vi "tsapp_transmit_canfd_sync.vi"(8 "error in (no error)":errorcluster, 9 "ATimeoutMS":i32, 10 "TCANFD":T1 {"ADLC" items=["0", "1", "2", "3", "4", "5", "6", "7", "8", "12", "16", "20", "24", "32", "48", "64"]; "AIsData" items=["Data Frame", "Remote Frame"]; "AIsStd" items=["标准帧", "扩展帧"]; "AId" format="%x"; "AIdxchn" items=["CHN1", "CHN2", "CHN3", "CHN4", "CHN5", "CHN6", "CHN7", "CHN8", "CHN9", "CHN10", "CHN11", "CHN12", "CHN13", "CHN14", "CHN15", "CHN16", "CHN17", "CHN18", "CHN19", "CHN20", "CHN21", "CHN22", "CHN23", "CHN24", "CHN25", "CHN26", "CHN27", "CHN28", "CHN29", "CHN30", "CHN31", "CHN32"]}, 11 "Path":path) -> (0 "error out":errorcluster, 2 "return":i32, 3 "Path output":path)   [LabVIEW 2014]
doc: "Function Introduction :\nSend CANFD message and only exit this function after detecting successful transmission. This function returns success,\nThe CANFD message must have been successfully sent to the CAN bus.\nCall location :\nSend CANFD message\nlimitations\nBecause this function requires deep support for device APIs, currently only TS supports this function interface\nAnd Vector series devices.\ninput parameter :\nACANFD: CANFD data packet. Please refer to chapter: TLIBCANFD: CANFD for the composition of TLIBCANFD data\nData type.\nATimeoutMS: timeout (milliseconds)\nReturn value :\n==0: Sent successfully\nOther values: Sending failed, please refer to the error code for the reason of the failure"
uses:
  Typedef/TLibCANFD_Interface.ctl
  Typedef/TLibCANFD.ctl
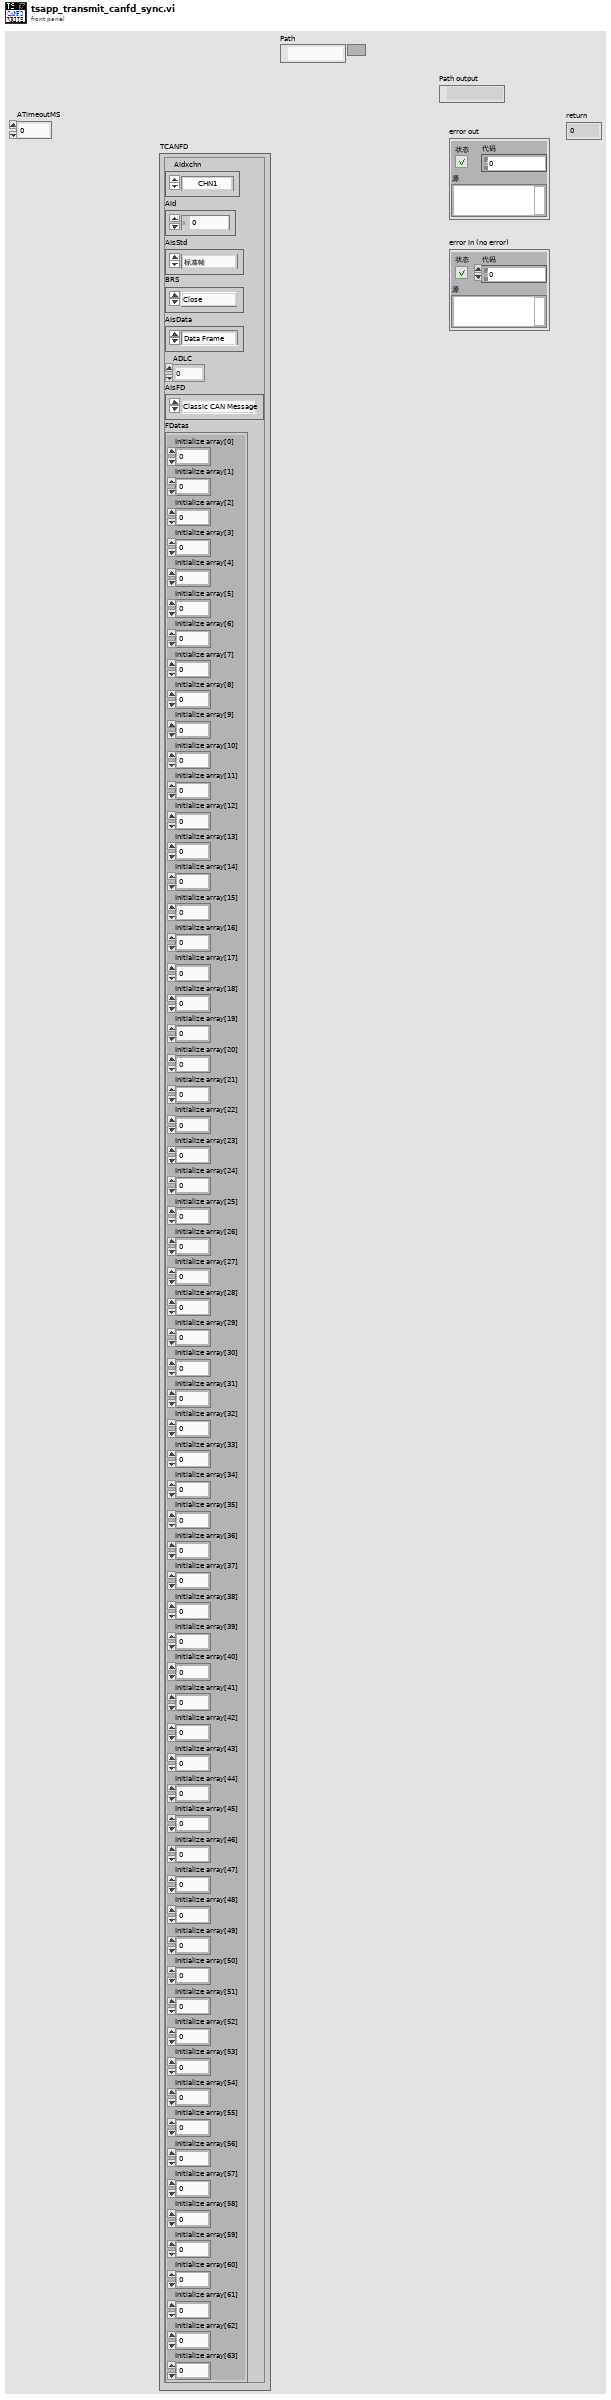
[diagram p1: front panel]
types:
  T1 = typedef "TLibCANFD.ctl" = cluster{"AIdxchn":u8, "AId":i32, "AIsStd":u8, "BRS":enum16{"Close", "Open"}, "AIsData":u8, "ADLC":i32, "AIsFD":enum16{"Classic CAN Message", "FD CAN Message"}, "FDatas":cluster{"Initialize array[0]":u8, "Initialize array[1]":u8, "Initialize array[2]":u8, "Initialize array[3]":u8, "Initialize array[4]":u8, "Initialize array[5]":u8, "Initialize array[6]":u8, "Initialize array[7]":u8, "Initialize array[8]":u8, "Initialize array[9]":u8, "Initialize array[10]":u8, "Initialize array[11]":u8, "Initialize array[12]":u8, "Initialize array[13]":u8, "Initialize array[14]":u8, "Initialize array[15]":u8, "Initialize array[16]":u8, "Initialize array[17]":u8, "Initialize array[18]":u8, "Initialize array[19]":u8, "Initialize array[20]":u8, "Initialize array[21]":u8, "Initialize array[22]":u8, "Initialize array[23]":u8, "Initialize array[24]":u8, "Initialize array[25]":u8, "Initialize array[26]":u8, "Initialize array[27]":u8, "Initialize array[28]":u8, "Initialize array[29]":u8, "Initialize array[30]":u8, "Initialize array[31]":u8, "Initialize array[32]":u8, "Initialize array[33]":u8, "Initialize array[34]":u8, "Initialize array[35]":u8, "Initialize array[36]":u8, "Initialize array[37]":u8, "Initialize array[38]":u8, "Initialize array[39]":u8, "Initialize array[40]":u8, "Initialize array[41]":u8, "Initialize array[42]":u8, "Initialize array[43]":u8, "Initialize array[44]":u8, "Initialize array[45]":u8, "Initialize array[46]":u8, "Initialize array[47]":u8, "Initialize array[48]":u8, "Initialize array[49]":u8, "Initialize array[50]":u8, "Initialize array[51]":u8, "Initialize array[52]":u8, "Initialize array[53]":u8, "Initialize array[54]":u8, "Initialize array[55]":u8, "Initialize array[56]":u8, "Initialize array[57]":u8, "Initialize array[58]":u8, "Initialize array[59]":u8, "Initialize array[60]":u8, "Initialize array[61]":u8, "Initialize array[62]":u8, "Initialize array[63]":u8}}
  T2 = typedef "TLibCANFD_Interface.ctl" = cluster{"FIdxChn":u8, "FProperties":u8, "FDLC":u8, "FFDProperties":u8, "FIdentifier":i32, "FTimeUS":u64, "FData":cluster{"[0]":u8, "[1]":u8, "[2]":u8, "[3]":u8, "[4]":u8, "[5]":u8, "[6]":u8, "[7]":u8, "[8]":u8, "[9]":u8, "[10]":u8, "[11]":u8, "[12]":u8, "[13]":u8, "[14]":u8, "[15]":u8, "[16]":u8, "[17]":u8, "[18]":u8, "[19]":u8, "[20]":u8, "[21]":u8, "[22]":u8, "[23]":u8, "[24]":u8, "[25]":u8, "[26]":u8, "[27]":u8, "[28]":u8, "[29]":u8, "[30]":u8, "[31]":u8, "[32]":u8, "[33]":u8, "[34]":u8, "[35]":u8, "[36]":u8, "[37]":u8, "[38]":u8, "[39]":u8, "[40]":u8, "[41]":u8, "[42]":u8, "[43]":u8, "[44]":u8, "[45]":u8, "[46]":u8, "[47]":u8, "[48]":u8, "[49]":u8, "[50]":u8, "[51]":u8, "[52]":u8, "[53]":u8, "[54]":u8, "[55]":u8, "[56]":u8, "[57]":u8, "[58]":u8, "[59]":u8, "[60]":u8, "[61]":u8, "[62]":u8, "[63]":u8}}
  T3 = cluster{"Initialize array[0]":u8, "Initialize array[1]":u8, "Initialize array[2]":u8, "Initialize array[3]":u8, "Initialize array[4]":u8, "Initialize array[5]":u8, "Initialize array[6]":u8, "Initialize array[7]":u8, "Initialize array[8]":u8, "Initialize array[9]":u8, "Initialize array[10]":u8, "Initialize array[11]":u8, "Initialize array[12]":u8, "Initialize array[13]":u8, "Initialize array[14]":u8, "Initialize array[15]":u8, "Initialize array[16]":u8, "Initialize array[17]":u8, "Initialize array[18]":u8, "Initialize array[19]":u8, "Initialize array[20]":u8, "Initialize array[21]":u8, "Initialize array[22]":u8, "Initialize array[23]":u8, "Initialize array[24]":u8, "Initialize array[25]":u8, "Initialize array[26]":u8, "Initialize array[27]":u8, "Initialize array[28]":u8, "Initialize array[29]":u8, "Initialize array[30]":u8, "Initialize array[31]":u8, "Initialize array[32]":u8, "Initialize array[33]":u8, "Initialize array[34]":u8, "Initialize array[35]":u8, "Initialize array[36]":u8, "Initialize array[37]":u8, "Initialize array[38]":u8, "Initialize array[39]":u8, "Initialize array[40]":u8, "Initialize array[41]":u8, "Initialize array[42]":u8, "Initialize array[43]":u8, "Initialize array[44]":u8, "Initialize array[45]":u8, "Initialize array[46]":u8, "Initialize array[47]":u8, "Initialize array[48]":u8, "Initialize array[49]":u8, "Initialize array[50]":u8, "Initialize array[51]":u8, "Initialize array[52]":u8, "Initialize array[53]":u8, "Initialize array[54]":u8, "Initialize array[55]":u8, "Initialize array[56]":u8, "Initialize array[57]":u8, "Initialize array[58]":u8, "Initialize array[59]":u8, "Initialize array[60]":u8, "Initialize array[61]":u8, "Initialize array[62]":u8, "Initialize array[63]":u8}
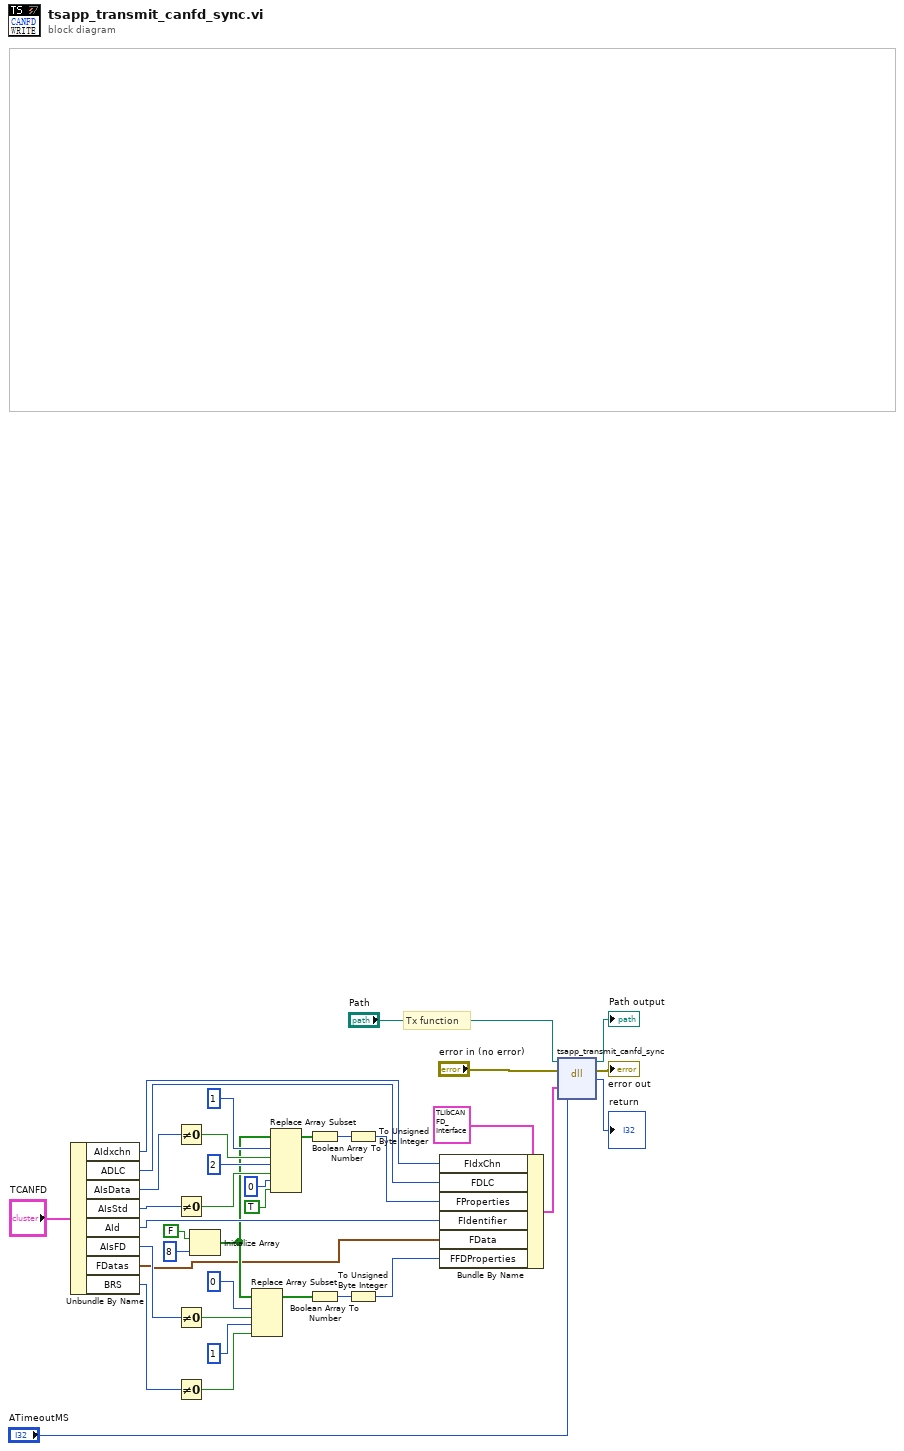
[diagram p0: block diagram]
diagram:
  # "Tx function"
  n1 = Unbundle By Name("TCANFD") -> ("AIdxchn"=w29:u8, "ADLC"=w20:i32, "AIsData"=w28:u8, "AIsStd"=w27:u8, "AId"=w30:i32, "AIsFD"=w15:enum16{"Classic CAN Message", "FD CAN Message"}, "FDatas"=w3:T3, "BRS"=w5:enum16{"Close", "Open"})
  n2 = Not Equal To 0?(x=w28) -> (x != 0?=w25:bool)
  n3 = Not Equal To 0?(x=w27) -> (x != 0?=w23:bool)
  n4 = Not Equal To 0?(x=w15) -> (x != 0?=w14:bool)
  n5 = Not Equal To 0?(x=w5) -> (x != 0?=w4:bool)
  n6 = Initialize Array(FALSE, 8 ("维数大小")) -> (w9:bool[])
  n7 = Replace Array Subset(array=w9, new element #1=w14, index #1=0 ("索引"), new element #2=w4, index #2=1 ("索引")) -> (w16:bool[])
  n8 = Replace Array Subset(array=w9, new element #1=w25, index #1=1 ("索引"), new element #2=w23, index #2=2 ("索引"), new element #3=TRUE ("新元素/子数组"), index #3=0 ("索引")) -> (w22:bool[])
  n9 = Boolean Array To Number(Boolean array=w22) -> (number=w21:u32)
  n10 = Boolean Array To Number(Boolean array=w16) -> (number=w17:u32)
  n11 = To Unsigned Byte Integer(number=w21) -> (unsigned 8bit integer=w19:u8)
  n12 = To Unsigned Byte Integer(number=w17) -> (unsigned 8bit integer=w12:u8)
  n13 = Bundle By Name(cluster=T2 {"FIdxChn"=0, "FProperties"=0, "FDLC"=0, "FFDProperties"=0, "FIdentifier"=0, "FTimeUS"=0, "FData"={"[0]"=0, "[1]"=0, "[2]"=0, "[3]"=0, "[4]"=0, "[5]"=0, "[6]"=0, "[7]"=0, "[8]"=0, "[9]"=0, "[10]"=0, "[11]"=0, "[12]"=0, "[13]"=0, "[14]"=0, "[15]"=0, "[16]"=0, "[17]"=0, "[18]"=0, "[19]"=0, "[20]"=0, "[21]"=0, "[22]"=0, "[23]"=0, "[24]"=0, "[25]"=0, "[26]"=0, "[27]"=0, "[28]"=0, "[29]"=0, "[30]"=0, "[31]"=0, "[32]"=0, "[33]"=0, "[34]"=0, "[35]"=0, "[36]"=0, "[37]"=0, "[38]"=0, "[39]"=0, "[40]"=0, "[41]"=0, "[42]"=0, "[43]"=0, "[44]"=0, "[45]"=0, "[46]"=0, "[47]"=0, "[48]"=0, "[49]"=0, "[50]"=0, "[51]"=0, "[52]"=0, "[53]"=0, "[54]"=0, "[55]"=0, "[56]"=0, "[57]"=0, "[58]"=0, "[59]"=0, "[60]"=0, "[61]"=0, "[62]"=0, "[63]"=0}} ("TLIBCANFD"), "FIdxChn"=w29, "FDLC"=w20, "FProperties"=w19, "FIdentifier"=w30, "FData"=w3, "FFDProperties"=w12) -> (w32:T2)
  n14 = dll-call lib="D:/Program Files (x86)/TOSUN/TSMaster/bin/TSMaster.dll" fn="tsapp_transmit_canfd_sync"(path in="Path", error in="error in (no error)", "ACAN"=w32, "ATimeoutMS"="ATimeoutMS") -> (path out=→"Path output":path, error out=→"error out":errorcluster, "tsapp_transmit_can_async"=→"return":i32)  [unwired: 3 in]
